vi "Configure Source to Single-Ganged.vi"(8 "error in":errorcluster, 10 "measurement configuration":T6 {"Measurement timeout" format="%.3p"; "Load device voltage/current rating" format="%#_6pA"; "Load output function" items=["DC Voltage"=1006, "DC Current"=1007, "Pulse Voltage"=1049, "Pulse Current"=1050]; "Power ON/Source output function" items=["DC Voltage"=1006, "DC Current"=1007, "Pulse Voltage"=1049, "Pulse Current"=1050]; "Load sense" items=["Local"=1008, "Remote"=1009]; "Load transient response" items=["Slow"=1041, "Normal"=1038, "Fast"=1039, "Custom"=1042]; "Power ON/Source sense" items=["Local"=1008, "Remote"=1009]; "Source transient response" items=["Slow"=1041, "Normal"=1038, "Fast"=1039, "Custom"=1042]; "Measurement duration" format="%.3p"; "Aperture time" format="%.3p"; "Load current/voltage limit high" format="%#_6p"; "Load current/voltage limit low" format="%#_6p"; "Load current/voltage limit range" format="%#_6p"; "Load voltage/current level range" format="%#_6p"; "Load voltage/current level" format="%#_6p"; "Source current/voltage limit high" format="%#_6p"; "Source current/voltage limit low" format="%#_6p"; "Power ON/Source current/voltage limit range" format="%#_6p"; "Source voltage/current level range" format="%#_6p"; "Power ON/Source voltage/current level" format="%#_6p"}, 11 "Single Point Perform Measurement in":T1) -> (0 "error out":errorcluster, 3 "Single Point Perform Measurement out":T1)   [LabVIEW 2021, in "Single Point_Channel Ganging.lvlib"]
uses:
  Single Point_Channel Ganging.lvlib
  <instrlib>/niDCPower/nidcpower.llb/niDCPower Source Mode.ctl
  Measurement Results.ctl
  shared subVIs/ctl/NIDCPower_channel_ganging - ctl - ganged config.ctl
  shared subVIs/ctl/NIDCPower_channel_ganging - ctl - channel mode.ctl
  shared subVIs/ctl/NIDCPower_channel_ganging - ctl - ganged session.ctl
  Controls/Perform measurement-control.ctl
  Measurement Configuration.ctl
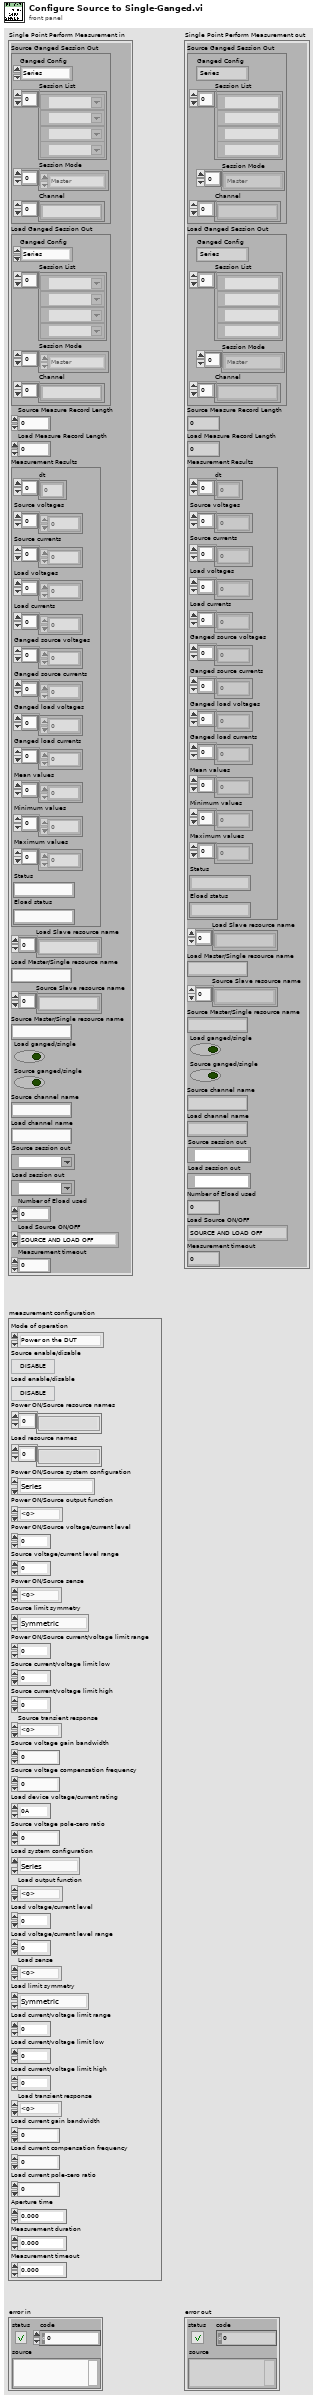
[diagram p1: front panel]
types:
  T1 = typedef "Single Point_Channel Ganging.lvlib/Perform measurement-control.ctl" = cluster{"Source Ganged Session Out":T2, "Load Ganged Session Out":T2, "Source Measure Record Length":i32, "Load Measure Record Length":i32, "Measurement Results":T5, "Load Slave resource name":string[], "Load Master/Single resource name":string, "Source Slave resource name":string[], "Source Master/Single resource name":string, "Load ganged/single":bool, "Source ganged/single":bool, "Source channel name":string, "Load channel name":string, "Source session out":refnum<k15>, "Load session out":refnum<k15>, "Number of Eload used":i32, "Load Source ON/OFF":enum16{"SOURCE AND LOAD OFF", "SOURCE ON", "LOAD ON", "SOURCE AND LOAD ON"}, "Measurement timeout":dbl}
  T2 = typedef "NIDCPower_channel_ganging - ctl - ganged session.ctl" = cluster{"Ganged Config":T3, "Session List":refnum<k15>[], "Session Mode":T4[], "Channel":string[]}
  T3 = typedef "NIDCPower_channel_ganging - ctl - ganged config.ctl" = enum32{"Series", "Parallel", "Manual"}
  T4 = typedef "NIDCPower_channel_ganging - ctl - channel mode.ctl" = enum32{"Master", "Slave", "Slave - Inverted"}
  T5 = typedef "Single Point_Channel Ganging.lvlib/Measurement Results.ctl" = cluster{"dt":dbl[], "Source voltages":dbl[], "Source currents":dbl[], "Load voltages":dbl[], "Load currents":dbl[], "Ganged source voltages":dbl[], "Ganged source currents":dbl[], "Ganged load voltages":dbl[], "Ganged load currents":dbl[], "Mean values":dbl[], "Minimum values":dbl[], "Maximum values":dbl[], "Status":string, "Eload status":string}
  T6 = typedef "Single Point_Channel Ganging.lvlib/Measurement Configuration.ctl" = cluster{"Mode of operation":enum32{"Power on the DUT", "Perform measurement", "Power off the DUT"}, "Source enable/disable":bool, "Load enable/disable":bool, "Power ON/Source resource names":string[], "Load resource names":string[], "Power ON/Source system configuration":enum32{"Series", "Parallel", "Manual"}, "Power ON/Source output function":i32, "Power ON/Source voltage/current level":dbl, "Source voltage/current level range":dbl, "Power ON/Source sense":i32, "Source limit symmetry":enum32{"Symmetric", "Asymmetric"}, "Power ON/Source current/voltage limit range":dbl, "Source current/voltage limit low":dbl, "Source current/voltage limit high":dbl, "Source transient response":i32, "Source voltage gain bandwidth":dbl, "Source voltage compensation frequency":dbl, "Load device voltage/current rating":dbl, "Source voltage pole-zero ratio":dbl, "Load system configuration":enum32{"Series", "Parallel", "Manual"}, "Load output function":i32, "Load voltage/current level":dbl, "Load voltage/current level range":dbl, "Load sense":i32, "Load limit symmetry":enum32{"Symmetric", "Asymmetric"}, "Load current/voltage limit range":dbl, "Load current/voltage limit low":dbl, "Load current/voltage limit high":dbl, "Load transient response":i32, "Load current gain bandwidth":dbl, "Load current compensation frequency":dbl, "Load current pole-zero ratio":dbl, "Aperture time":dbl, "Measurement duration":dbl, "Measurement timeout":dbl}
  T7 = typedef "niDCPower Source Mode.ctl" = i32
  T8 = typedef "NIDCPower_channel_ganging - ctl - channel def.ctl" = cluster{"resource name":refnum<k15>, "channels":string, "Channel Mode":T4}
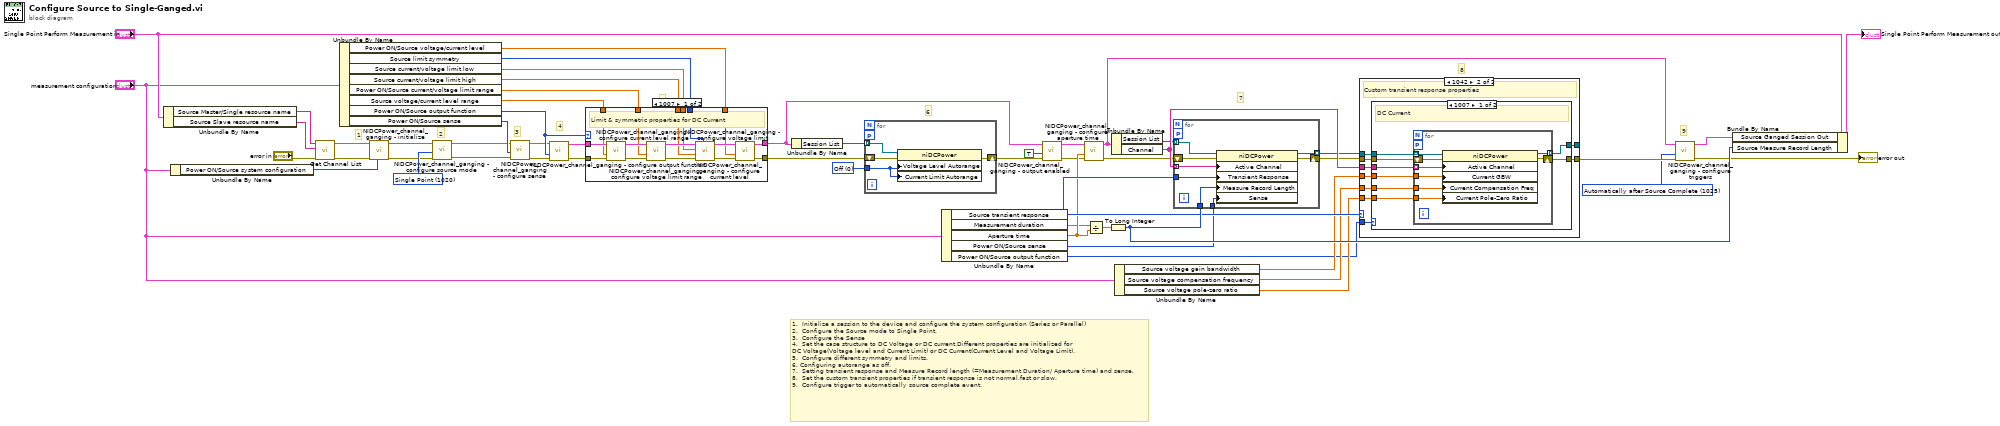
[diagram p0: block diagram]
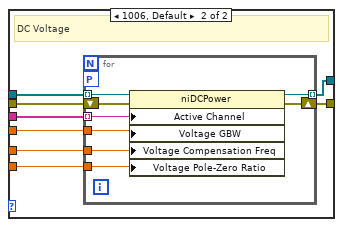
[diagram p3: hidden frame]
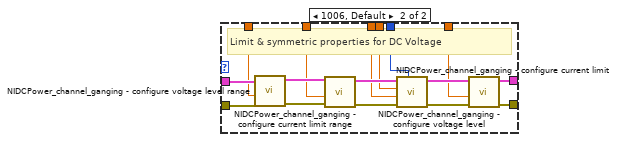
[diagram p4: hidden frame]
diagram:
  w36 = 1025 items=["Automatically after Source Complete"=1025, "On Demand"=1026, "On Measure Trigger"=1027] ("Measure When")
  w29 = 0 items=["Off", "On"] ("Source:DC Voltage:Voltage Level Autorange")
  w4 = T7 1020 items=["Single Point"=1020, "Sequence"=1021] ("source mode")
  # "9"
  # "8"
  # "7"
  # "6"
  # "5"
  # "4"
  # "3"
  # "2"
  # "1"
  # "1.  Initialize a session to the device and configure the system configuration (Series or Parallel)\n2.  Configure the Source mode to Single Point.\n3.  Configure the Sense\n4.  Set the case structure to DC Voltage or DC current.Different properties are initialized for \nDC Voltage(Voltage level and Current Limit) or DC Current(Current Level and Voltage Limit). \n5.  Configure different symmetry and limits.\n6. Configuring autorange as off.\n7.  Setting transient response and Measure Record length (=Measurement Duration/ Aperture time) and sense.\n8.  Set the custom transient properties if transient response is not normal,fast or slow.\n9.  Configure trigger to automatically source complete event."
  n1 = Unbundle By Name("Single Point Perform Measurement in") -> ("Source Master/Single resource name"=w22:string, "Source Slave resource name"=w23:string[])
  n2 = Unbundle By Name("measurement configuration") -> ("Power ON/Source system configuration"=w51:enum32{"Series", "Parallel", "Manual"})
  n3 = call "Get Channel List.vi"("error in (no error)"="error in", "Slave resource names"=w23, "Master resouce name"=w22) -> ("error out"=w25:errorcluster, "Channel List"=w21:T8[])  [unwired: 7 in]
  n4 = Unbundle By Name("measurement configuration") -> ("Power ON/Source voltage/current level"=w18:dbl, "Source limit symmetry"=w17:enum32{"Symmetric", "Asymmetric"}, "Source current/voltage limit low"=w16:dbl, "Source current/voltage limit high"=w15:dbl, "Power ON/Source current/voltage limit range"=w14:dbl, "Source voltage/current level range"=w6:dbl, "Power ON/Source output function"=w19:i32, "Power ON/Source sense"=w20:i32)
  n5 = call "NIDCPower_channel_ganging - initialize.vi"("Ganged Config"=w51, "error in (no error)"=w25, "Channel List"=w21) -> ("error out"=w3:errorcluster, "Ganged Session Out"=w2:T2)  [unwired: 7 in]
  n6 = call "NIDCPower_channel_ganging - configure source mode.vi"("error in (no error)"=w3, "source mode"=w4, "Ganged Session In"=w2) -> ("error out"=w8:errorcluster, "Ganged Session Out"=w7:T2)  [unwired: 7 in]
  n7 = call "NIDCPower_channel_ganging - configure sense.vi"("error in (no error)"=w8, "sense"=w20, "Ganged Session In"=w7) -> ("error out"=w10:errorcluster, "Ganged Session Out"=w9:T2)  [unwired: 7 in]
  n8 = call "NIDCPower_channel_ganging - configure output function.vi"("error in (no error)"=w10, "output function"=w19, "Ganged Session In"=w9) -> ("error out"=w12:errorcluster, "Ganged Session Out"=w11:T2)  [unwired: 7 in]
  n9 = case shown="1007" w19 {
    tunnel: w6 -> [w60 w76]
    tunnel: w14 -> [w59 w75]
    tunnel: w15 -> [w58 w74]
    tunnel: w16 -> [w57 w73]
    tunnel: w17 -> [w56 w72]
    tunnel: w11 -> [w70 w80]
    tunnel: w12 -> [w69 w79]
    tunnel: [w61 w78] -> w26
    tunnel: [w62 w77] -> w13
    tunnel: w18 -> [w55 w71]
    frame 1007 {
      # "Limit & symmetric properties for DC Current"
      n10 = call "NIDCPower_channel_ganging - configure current level range.vi"("error in (no error)"=w69, "current level range"=w60, "Ganged Session In"=w70) -> ("error out"=w67:errorcluster, "Ganged Session Out"=w68:T2)  [unwired: 7 in]
      n11 = call "NIDCPower_channel_ganging - configure voltage limit range.vi"("error in (no error)"=w67, "voltage level range"=w59, "Ganged Session In"=w68) -> ("error out"=w65:errorcluster, "Ganged Session Out"=w66:T2)  [unwired: 7 in]
      n12 = call "NIDCPower_channel_ganging - configure voltage limit.vi"("Limit Symmetry"=w56, "error in (no error)"=w65, "voltage limit/hi"=w58, "voltage limit lo"=w57, "Ganged Session In"=w66) -> ("error out"=w63:errorcluster, "Ganged Session Out"=w64:T2)  [unwired: 5 in]
      n13 = call "NIDCPower_channel_ganging - configure current level.vi"("error in (no error)"=w63, "current level"=w55, "Ganged Session In"=w64) -> ("error out"=w61:errorcluster, "Ganged Session Out"=w62:T2)  [unwired: 7 in]
    }
    frame 1006, Default {
      # "Limit & symmetric properties for DC Voltage"
      n14 = call "NIDCPower_channel_ganging - configure voltage level range.vi"("error in (no error)"=w79, "voltage level range"=w76, "Ganged Session In"=w80) -> ("error out"=w83:errorcluster, "Ganged Session Out"=w86:T2)  [unwired: 7 in]
      n15 = call "NIDCPower_channel_ganging - configure current limit range.vi"("error in (no error)"=w83, "current limit range"=w75, "Ganged Session In"=w86) -> ("error out"=w82:errorcluster, "Ganged Session Out"=w85:T2)  [unwired: 7 in]
      n16 = call "NIDCPower_channel_ganging - configure current limit.vi"("Limit Symmetry"=w72, "error in (no error)"=w82, "Current limit/hi"=w74, "Current limit lo"=w73, "Ganged Session In"=w85) -> ("error out"=w81:errorcluster, "Ganged Session Out"=w84:T2)  [unwired: 5 in]
      n17 = call "NIDCPower_channel_ganging - configure voltage level.vi"("error in (no error)"=w81, "voltage level"=w71, "Ganged Session In"=w84) -> ("error out"=w78:errorcluster, "Ganged Session Out"=w77:T2)  [unwired: 7 in]
    }
  }
  n18 = Unbundle By Name(w13) -> ("Session List"=w27:refnum<k15>[])
  n19 = for {
    tunnel: w27 -> [w90] mode=indexing
    shift-right: [w88] -> w28
    shift-left: w26 -> [w89]
    workers-P: _ -> [_]
    tunnel: w29 -> [w87]
    n20 = property class="niDCPower"(reference=w90, error in=w89, "Voltage Level Autorange"=w87, "Current Limit Autorange"=w87) -> (error out=w88:errorcluster)  [unwired: 1 out]
  }
  n21 = Unbundle By Name("measurement configuration") -> ("Source transient response"=w49:i32, "Measurement duration"=w38:dbl, "Aperture time"=w40:dbl, "Power ON/Source sense"=w39:i32, "Power ON/Source output function"=w45:i32)
  n22 = call "NIDCPower_channel_ganging - output enabled.vi"("error in (no error)"=w28, "output enabled"=TRUE, "Ganged Session In"=w13) -> ("error out"=w31:errorcluster, "Ganged Session Out"=w32:T2)  [unwired: 7 in]
  n23 = call "NIDCPower_channel_ganging - configure aperture time.vi"("error in (no error)"=w31, "aperture time"=w40, "Ganged Session In"=w32) -> ("error out"=w30:errorcluster, "Ganged Session Out"=w53:T2)  [unwired: 7 in]
  n24 = Divide(x=w38, y=w40) -> (x/y=w37:dbl)
  n25 = To Long Integer(number=w37) -> (32bit integer=w54:i32)
  n26 = Unbundle By Name(w53) -> ("Session List"=w33:refnum<k15>[], "Channel"=w44:string[])
  n27 = Unbundle By Name("measurement configuration") -> ("Source voltage gain bandwidth"=w46:dbl, "Source voltage compensation frequency"=w48:dbl, "Source voltage pole-zero ratio"=w47:dbl)
  n28 = for {
    tunnel: [w98] -> w43 mode=indexing
    shift-right: [w96] -> w41
    shift-left: w30 -> [w97]
    workers-P: _ -> [_]
    tunnel: w33 -> [w95] mode=indexing
    tunnel: w49 -> [w92]
    tunnel: w39 -> [w94]
    tunnel: w54 -> [w93]
    tunnel: w44 -> [w91] mode=indexing
    n29 = property class="niDCPower"(reference=w95, error in=w97, "Active Channel"=w91, "Transient Response"=w92, "Measure Record Length"=w93, "Sense"=w94) -> (reference out=w98:refnum<k15>, error out=w96:errorcluster)
  }
  n30 = case shown="1042" w49 {
    tunnel: w41 -> [w100 w109]
    tunnel: [w100 w108] -> w42
    tunnel: w43 -> [w99 w107]
    tunnel: w44 -> [_ w106]
    tunnel: w45 -> [_ w105]
    tunnel: w46 -> [_ w104]
    tunnel: w47 -> [_ w103]
    tunnel: w48 -> [_ w102]
    tunnel: [w99 w101] -> _
    frame Default {
      # "For normal ,slow and fast transient response"
    }
    frame 1042 {
      # "Custom transient response properties"
      n31 = case shown="1007" w105 {
        tunnel: w109 -> [w117 w133]
        tunnel: [w116 w132] -> w108
        tunnel: w107 -> [w115 w131]
        tunnel: w106 -> [w113 w130]
        tunnel: w104 -> [w114 w129]
        tunnel: w103 -> [w111 w127]
        tunnel: w102 -> [w112 w128]
        tunnel: [w110 w126] -> w101
        frame 1007 {
          # "DC Current"
          n32 = for {
            workers-P: _ -> [_]
            shift-right: [w124] -> w116
            shift-left: w117 -> [w125]
            tunnel: w115 -> [w123] mode=indexing
            tunnel: [w122] -> w110 mode=indexing
            tunnel: w114 -> [w121]
            tunnel: w113 -> [w120] mode=indexing
            tunnel: w112 -> [w119]
            tunnel: w111 -> [w118]
            n33 = property class="niDCPower"(reference=w123, error in=w125, "Active Channel"=w120, "Current GBW"=w121, "Current Compensation Freq"=w119, "Current Pole-Zero Ratio"=w118) -> (reference out=w122:refnum<k15>, error out=w124:errorcluster)
          }
        }
        frame 1006, Default {
          # "DC Voltage"
          n34 = for {
            workers-P: _ -> [_]
            shift-right: [w134] -> w132
            shift-left: w133 -> [w141]
            tunnel: w131 -> [w140] mode=indexing
            tunnel: [w139] -> w126 mode=indexing
            tunnel: w130 -> [w138] mode=indexing
            tunnel: w129 -> [w137]
            tunnel: w128 -> [w136]
            tunnel: w127 -> [w135]
            n35 = property class="niDCPower"(reference=w140, error in=w141, "Active Channel"=w138, "Voltage GBW"=w137, "Voltage Compensation Freq"=w136, "Voltage Pole-Zero Ratio"=w135) -> (reference out=w139:refnum<k15>, error out=w134:errorcluster)
          }
        }
      }
    }
  }
  n36 = call "NIDCPower_channel_ganging - configure triggers.vi"("error in (no error)"=w42, "Measure When"=w36, "Ganged Session In"=w53) -> ("error out"=→"error out":errorcluster, "Ganged Session Out"=w35:T2)  [unwired: 7 in]
  n37 = Bundle By Name(cluster="Single Point Perform Measurement in", "Source Ganged Session Out"=w35, "Source Measure Record Length"=w54) -> (→"Single Point Perform Measurement out":T1)
